vi "onTestDiscovery.vi"(8 "error in (no error)":errorcluster, 11 "Unit Tests for Runner in":refnum<class "Unit Tests for Runner.lvclass">) -> (0 "error out":errorcluster, 2 "Test VIs":path[](array[path]), 3 "Unit Tests for Runner out":refnum<class "Unit Tests for Runner.lvclass">)   [LabVIEW 2013, in "Unit Tests for Runner.lvclass"]
uses:
  Unit Tests for Runner.lvclass
  Unit Tests for Runner.lvclass/Unit Tests for Runner.ctl
  classes/Test/Test.lvclass
  classes/Assert/Assert.lvclass
  classes/Test Runner/Test Runner.lvclass
  classes/Test Runner.Folder/Test Runner.Folder.lvclass
  classes/Test Runner.Collection/Test Runner.Collection.lvclass
panel:
  out "Pass?":bool
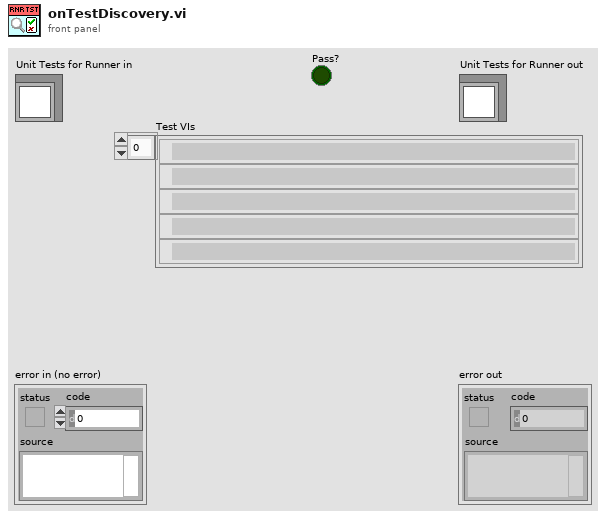
[diagram p1: front panel]
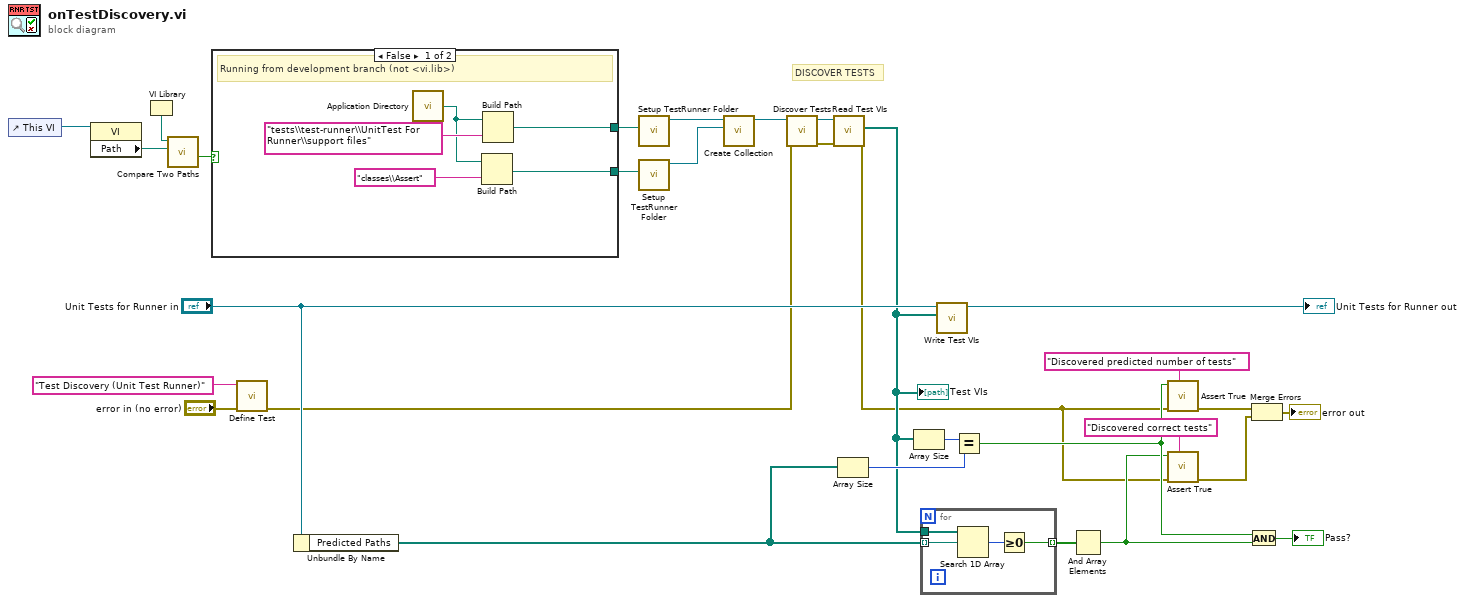
[diagram p0: block diagram]
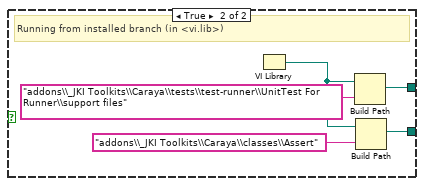
[diagram p2: hidden frame]
diagram:
  # "DISCOVER TESTS"
  n1 = control-ref of="This VI"() -> (w4:refnum<vi>)
  n2 = property on="Property Node" class="VI"(reference=w4) -> ("Path"=w3:path)  [unwired: 1 in, 2 out]
  n3 = VI Library() -> (path=w2:path)
  n4 = call <vilib>:"Compare Two Paths.vi"("Path 2"=w3, "Path 1"=w2) -> ("Path 2 Relative to Path 1?"=w1:bool)  [unwired: 6 in, 3 out]
  n5 = case shown="False" w1 {
    tunnel: [w34 w39] -> w15
    tunnel: [w32 w37] -> w10
    frame False {
      # "Running from development branch (not <vi.lib>)"
      n6 = call <vilib>:"Application Directory.vi"() -> ("Application Directory"=w31:path)
      n7 = Build Path(base path=w31, name or relative path="classes\\Assert") -> (appended path=w32:path)
      n8 = Build Path(base path=w31, name or relative path="tests\\test-runner\\UnitTest For Runner\\support files") -> (appended path=w34:path)
    }
    frame True {
      # "Running from installed branch (in <vi.lib>)"
      n9 = VI Library() -> (path=w36:path)
      n10 = Build Path(base path=w36, name or relative path="addons\\_JKI Toolkits\\Caraya\\tests\\test-runner\\UnitTest For Runner\\support files") -> (appended path=w39:path)
      n11 = Build Path(base path=w36, name or relative path="addons\\_JKI Toolkits\\Caraya\\classes\\Assert") -> (appended path=w37:path)
    }
  }
  n12 = call "Define Test.vi"("error in (no error)"="error in (no error)", "Label (VI Title)"="Test Discovery (Unit Test Runner)" ("name or relative path")) -> ("error out"=w9:errorcluster)  [unwired: 9 in]
  n13 = Unbundle By Name("Unit Tests for Runner in") -> ("Predicted Paths"=w19:path[])
  n14 = call "Setup TestRunner Folder.vi"("Directory to search"=w15) -> ("Test Runner.Folder out"=w8:refnum<class "Test Runner.Folder.lvclass">)  [unwired: 9 in, 1 out]
  n15 = call "Setup TestRunner Folder.vi"("Directory to search"=w10) -> ("Test Runner.Folder out"=w7:refnum<class "Test Runner.Folder.lvclass">)  [unwired: 9 in, 1 out]
  n16 = call "Create Collection.vi"("Test Runner 2"=w7, "Test Runner 1"=w8) -> ("Test Runner.Collection out"=w6:refnum<class "Test Runner.Collection.lvclass">)  [unwired: 8 in, 1 out]
  n17 = call "Discover Tests.vi"("error in (no error)"=w9, "Test Runner in"=w6) -> ("error out"=w12:errorcluster, "Test Runner out"=w14:refnum<class "Test Runner.Collection.lvclass">)  [unwired: 8 in]
  n18 = call "Read Test VIs.vi"("error in (no error)"=w12, "Test Runner in"=w14) -> ("error out"=w11:errorcluster, "Test VIs"=w13:path[])  [unwired: 7 in, 1 out]
  "Test VIs" <- w13
  n19 = Array Size(array=w19) -> (size(s)=w18:i32)
  n20 = Array Size(array=w13) -> (size(s)=w29:i32)
  n21 = for {
    tunnel: w13 -> [w44]
    tunnel: [w42] -> w21 mode=indexing
    tunnel: w19 -> [w41] mode=indexing
    n22 = Search 1D Array(1D array=w44, element=w41) -> (index of element=w43:i32)  [unwired: 1 in]
    n23 = Greater Or Equal To 0?(x=w43) -> (x >= 0?=w42:bool)
  }
  n24 = call "Write Test VIs.vi"("Test VIs"=w13, "Test Runner in"="Unit Tests for Runner in") -> ("Test Runner out"=→"Unit Tests for Runner out":refnum<class "Unit Tests for Runner.lvclass">)  [unwired: 8 in, 1 out]
  n25 = Equal?(x=w29, y=w18) -> (x = y?=w25:bool)
  n26 = And Array Elements(Boolean array=w21) -> (logical AND=w20:bool)
  n27 = call "Assert True.vi"("Label"="Discovered predicted number of tests", "error in (no error)"=w11, "True?"=w25) -> ("error out"=w28:errorcluster)  [unwired: 8 in]
  n28 = call "Assert True.vi"("Label"="Discovered correct tests", "error in (no error)"=w11, "True?"=w20) -> ("error out"=w27:errorcluster)  [unwired: 8 in]
  n29 = And(x=w25, y=w20) -> (x .and. y?=→"Pass?":bool)
  n30 = Merge Errors(w28, w27) -> (→"error out":errorcluster)
